vi "Set FP size.vi"(8 "error in (no error)":errorcluster, 9 "Height":i16, 10 "Width":i16, 11 "VI Refnum":refnum<vi>) -> (0 "error out":errorcluster, 3 "VI Refnum out":refnum<vi>)   [LabVIEW 2011, in "COSYLib.lvlib"]
uses:
  COSYLib.lvlib
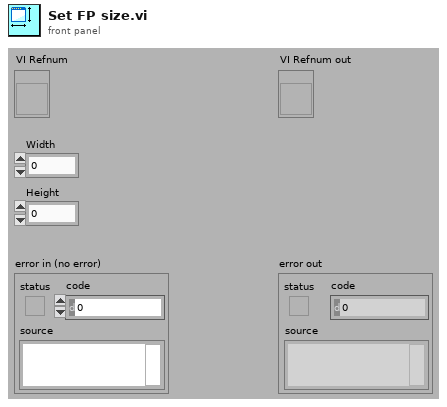
[diagram p1: front panel]
types:
  T1 = typedef "LVRectTypeDef.ctl" = cluster{"left":i16, "top":i16, "right":i16, "bottom":i16}
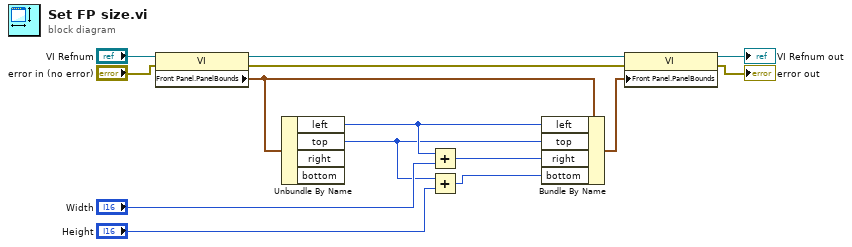
[diagram p0: block diagram]
diagram:
  n1 = property class="VI"(reference="VI Refnum", error in="error in (no error)") -> (reference out=w11:refnum<vi>, error out=w8:errorcluster, "Front Panel.PanelBounds"=w13:T1)
  n2 = Unbundle By Name(w13) -> ("left"=w6:i16, "top"=w1:i16)  [unwired: 2 out]
  n3 = Add(x=w6, y="Width") -> (x+y=w4:i16)
  n4 = Add(x=w1, y="Height") -> (x+y=w3:i16)
  n5 = Bundle By Name(cluster=w13, "left"=w6, "top"=w1, "right"=w4, "bottom"=w3) -> (w12:T1)
  n6 = property class="VI"(reference=w11, error in=w8, "Front Panel.PanelBounds"=w12) -> (reference out=→"VI Refnum out":refnum<vi>, error out=→"error out":errorcluster)
